vi "FlexDDS-NG_DCP_Command.vi"(9 "command string":string="update:u", 10 "Channels":T1(ring)=enum."Both channels", 11 "initial instruction string":string) -> (3 "appended instruction string":string="dcp update:u\r")   [LabVIEW 2016]
panel:
  # "Send raw 48 bit instruction"
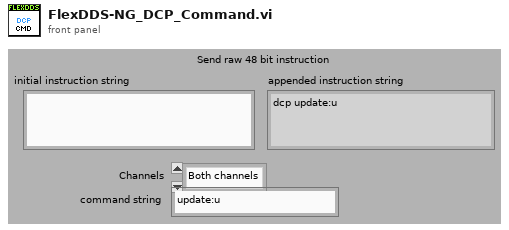
[diagram p1: front panel]
types:
  T1 = enum32{"Channel 0", "Channel 1", "Both channels"}
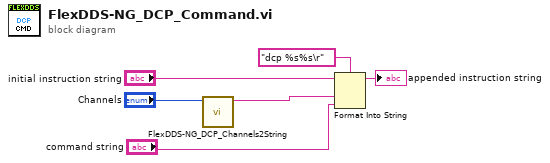
[diagram p0: block diagram]
diagram:
  n1 = call "FlexDDS-NG_DCP_Channels2String.vi"("Channels"="Channels") -> ("channels string"=w2:string)  [unwired: 10 in]
  n2 = Format Into String(format string="dcp %s%s\r", initial string="initial instruction string", w2, "command string") -> (resulting string=→"appended instruction string":string)  [unwired: 1 in, 1 out]
